vi "LiftControl.vi"(8 "error in":errorcluster) -> ()   [LabVIEW 2014]
uses:
  <vilib>/Rock Robotics/WPI/Joystick/WPI_JoystickGetSetRefNum.vi
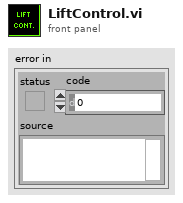
[diagram p1: front panel]
types:
  T1 = typedef "WPI_JoystickDevRef.ctl" = cluster{"Device":T2}
  T2 = typedef "WPI_JoystickDeviceEnum.ctl" = enum16{"USB 0", "USB 1", "USB 2", "USB 3", "USB 4", "USB 5"}
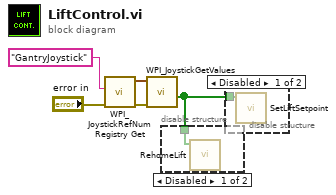
[diagram p0: block diagram]
diagram:
  n1 = call <vilib>:"WPI_JoystickRefNum Registry Get.vi"("error in (no error)"="error in", "refnum name"="GantryJoystick") -> ("error out"=w3:errorcluster, "JoystickDevRef"=w4:T1)  [unwired: 8 in]
  n2 = call <vilib>:"WPI_JoystickGetValues.vi"("error in (no error)"=w3, "JoystickDevRef"=w4) -> ("Buttons"=w1:bool[])  [unwired: 5 in, 4 out]
  n3 = disable-structure shown="Disabled" {
    disable-tunnel: w1 -> [w6 _]
    frame Disabled {
      n4 = call "RehomeLift.vi"("array"=w6) -> ()  [unwired: 11 in]
    }
    frame Enabled {
    }
  }
  n5 = disable-structure shown="Disabled" {
    disable-tunnel: w1 -> [w7 _]
    frame Disabled {
      n6 = call "SetLiftSetpoint.vi"("Buttons"=w7) -> ()  [unwired: 11 in]
    }
    frame Enabled {
    }
  }
